vi "MOKE1_jai.vi"() -> ()   [LabVIEW 2021]
uses:
  <vilib>/Analysis/NI_AALBase.lvlib
  <vilib>/Analysis/baseanly.llb/Mean (DBL).vi
  <vilib>/Analysis/Matrix/Datatypes/RealMatrix.ctl
  <vilib>/Analysis/Matrix/NI_Matrix.lvlib
panel:
  out "y_mat":T1
  in  "stop":bool
  in  "Total Loops":dbl
  out "Current Loop":i32
  in  "Time / Step":i64
  in  "Number of Samples":i32=100
  out "Graph For Photodiode":cluster{"Y":dbl[], "Y":dbl[]}[](graph)
  out "Photodiode Level":dbl
  out "Current Voltage":dbl
  in  "Scans From 0 to Max Voltage":i32
  in  "Voltage":dbl
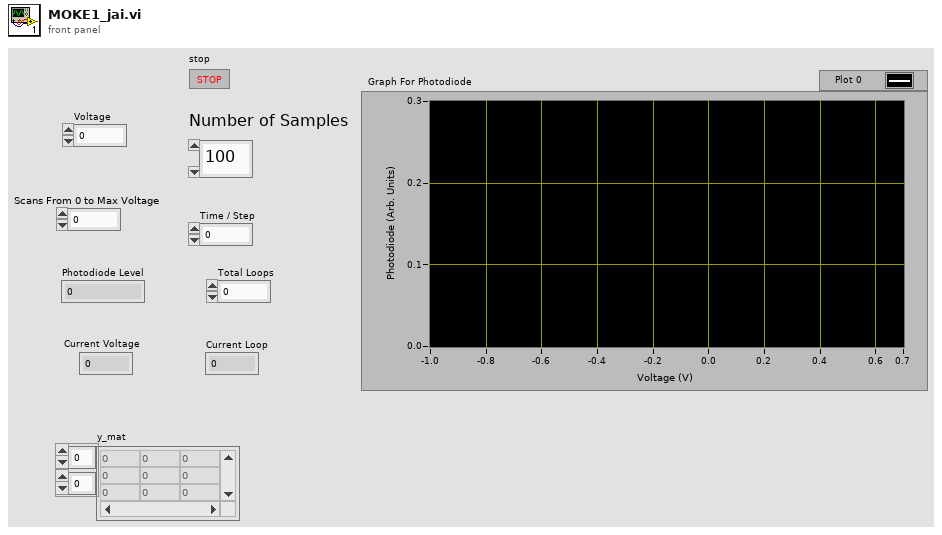
[diagram p1: front panel]
types:
  T1 = typedef "NI_Matrix.lvlib/RealMatrix.ctl" = dbl[][]
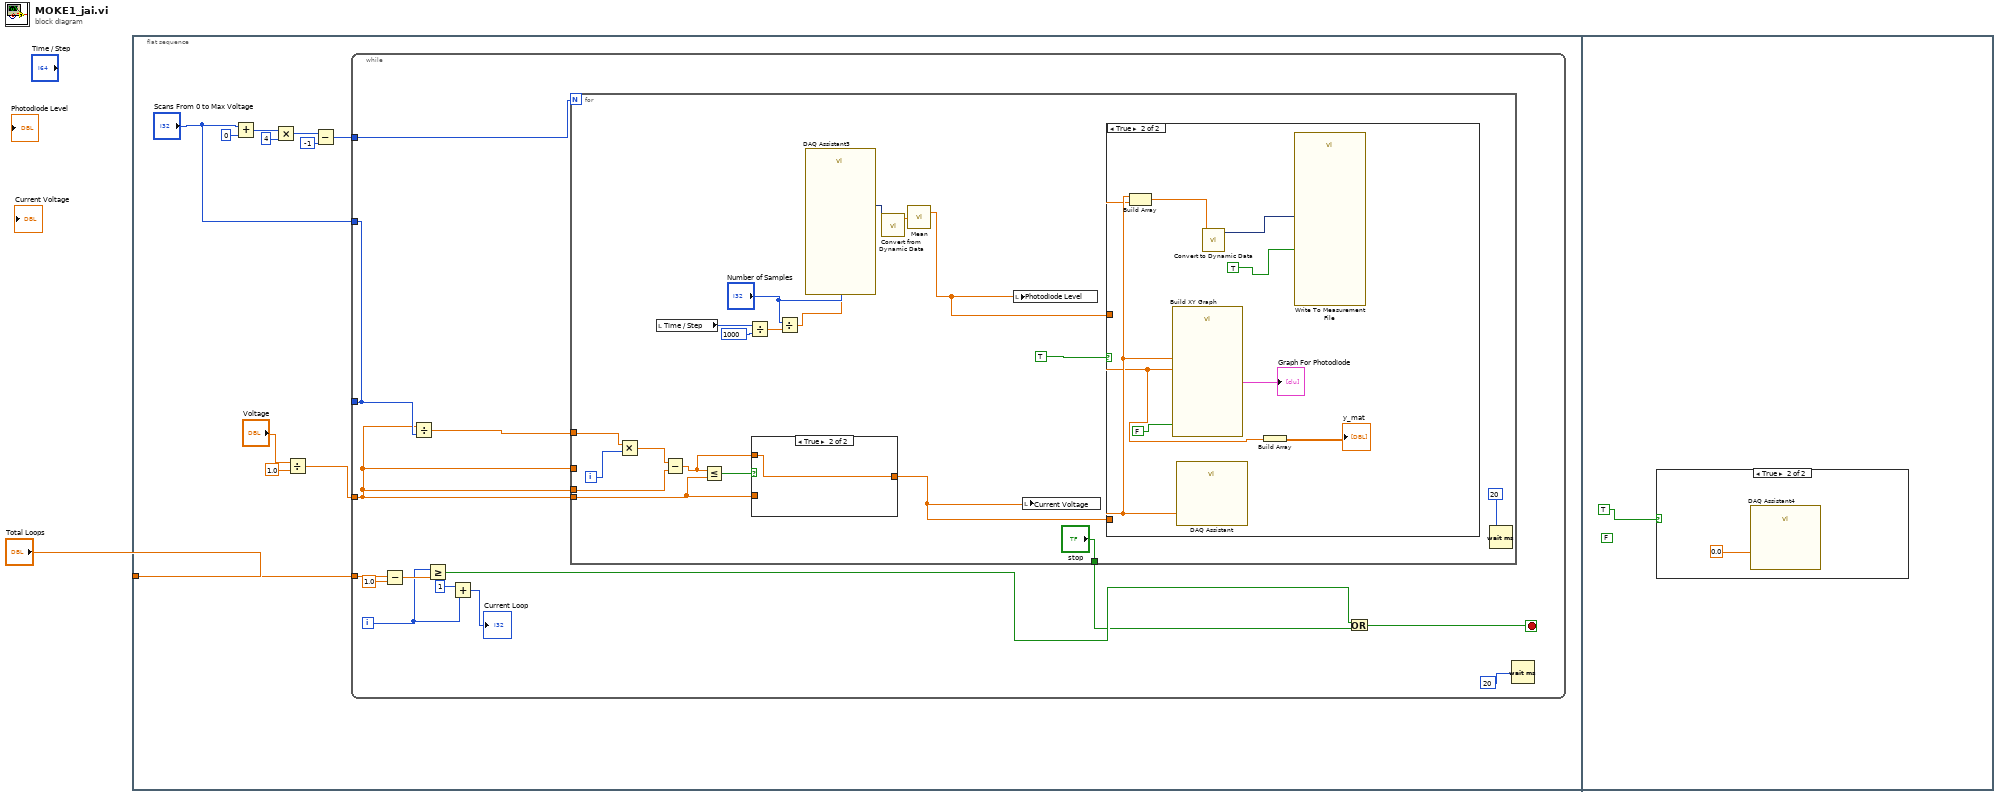
[diagram p0: block diagram]
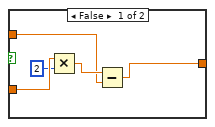
[diagram p2: hidden frame]
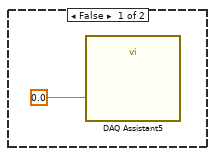
[diagram p4: hidden frame]
diagram:
  n1 = flat-sequence {
    tunnel: "Total Loops" -> [w5]
    frame #0 {
      n2 = Add(x="Scans From 0 to Max Voltage", y=0) -> (x+y=w11:i32)
      n3 = Multiply(x=w11, y=4) -> (x*y=w12:i32)
      n4 = Divide(x="Voltage", y=1.0) -> (x/y=w2:dbl)
      n5 = Subtract(x=w12, y=-1) -> (x-y=w7:i32)
      n6 = while {
        tunnel: w5 -> [w25]
        tunnel: [w15] -> _
        tunnel: w7 -> [w16]
        tunnel: "Scans From 0 to Max Voltage" -> [w15]
        tunnel: w2 -> [w13]
        i -> [w14]
        stop <- w18 stop-if-true
        n7 = Subtract(x=w25, y=1.0) -> (x-y=w24:dbl)
        n8 = Divide(x=w13, y=w15) -> (x/y=w26:dbl)
        n9 = Greater Or Equal?(x=w14, y=w24) -> (x >= y?=w19:bool)
        n10 = Add(x=1, y=w14) -> (x+y=→"Current Loop":i32)
        n11 = for {
          N: w16 -> [_]
          tunnel: w26 -> [w45]
          tunnel: w13 -> [_]
          tunnel: w13 -> [w42]
          tunnel: w13 -> [w38]
          tunnel: ["stop"] -> w17
          i -> [w27]
          n12 = Multiply(x=w45, y=w27) -> (x*y=w43:dbl)
          n13 = local read "Time / Step"() -> (w34:i64)
          n14 = Subtract(x=w43, y=w42) -> (x-y=w40:dbl)
          n15 = Less Or Equal?(x=w40, y=w38) -> (x <= y?=w41:bool)
          n16 = Divide(x=w34, y=i64 1000) -> (x/y=w35:dbl)
          n17 = case shown="True" w41 {
            tunnel: w40 -> [w47 w51]
            tunnel: [w46 w51] -> w39
            tunnel: w38 -> [w50 _]
            frame False {
              n18 = Multiply(x=w50, y=2) -> (x*y=w48:dbl)
              n19 = Subtract(x=w48, y=w47) -> (x-y=w46:dbl)
            }
            frame True {
            }
          }
          n20 = Divide(x="Number of Samples", y=w35) -> (x/y=w36:dbl)
          n21 = call "DAQ Assistant3"("rate"=w36, "number of samples"="Number of Samples") -> ("data"=w32:dynamicdata)  [unwired: 4 in, 13 out]
          n22 = call "Convert from Dynamic Data"("Dynamic Data Type"=w32) -> ("Array"=w31:dbl[])  [unwired: 3 in]
          n23 = call-poly <vilib>:"Mean.vi"("X"=w31) -> ("mean"=w30:dbl)  [unwired: 1 out]
          n24 = local write "Photodiode Level"(w30) -> ()
          n25 = local write "Current Voltage"(w39) -> ()
          n26 = case shown="True" TRUE {
            tunnel: w39 -> [_ w58]
            tunnel: w30 -> [_ w53]
            frame False {
            }
            frame True {
              n27 = Build Array(w58, w53) -> (w56:dbl[])
              n28 = call "Build XY Graph"("Reset"=FALSE, "Y Input"=w53, "X Input"=w58) -> ("XY Graph"=→"Graph For Photodiode":cluster{"X":dbl[], "Y":dbl[]}[])  [unwired: 7 in, 1 out]
              n29 = call "DAQ Assistant"("data"=w58) -> ()  [unwired: 17 in, 2 out]
              n30 = call "Convert to Dynamic Data"("Array"=w56) -> ("Dynamic Data Type"=w54:dynamicdata)  [unwired: 3 in]
              n31 = Build Array(w53) -> (→"y_mat":T1)
              n32 = call "Write To Measurement File"("Signals"=w54, "Enable"=TRUE) -> ()  [unwired: 15 in, 3 out]
            }
          }
          n33 = Wait (ms)(milliseconds to wait=20) -> ()  [unwired: 1 out]
        }
        n34 = Or(x=w19, y=w17) -> (x .or. y?=w18:bool)
        n35 = Wait (ms)(milliseconds to wait=u32 20) -> ()  [unwired: 1 out]
      }
    }
    frame #1 {
      (unwired) FALSE
      n36 = case shown="True" TRUE {
        frame False {
          n37 = call "DAQ Assistant5"("data"=0.0) -> ()  [unwired: 17 in, 2 out]
        }
        frame True {
          n38 = call "DAQ Assistant4"("data"=0.0) -> ()  [unwired: 17 in, 2 out]
        }
      }
    }
  }
